vi "Read Device ID Type1.vi"(8 "error in (no error)":errorcluster, 11 "device data model in":refnum<class "Standard Data Model1.lvclass">) -> (0 "error out":errorcluster, 2 "read device ID code":u8(ring)=1 items=["None"=0, "Basic Stream"=1, "Regular Stream"=2, "Extended Stream"=3, "Basic Stream/Individual"=129, "Regular Stream/Individual"=130, "Extended Stream/Individual"=131], 3 "device data model out":refnum<class "Standard Data Model1.lvclass">)   [LabVIEW 2019, in "NI_modbus_upd.lvlib" / "Standard Data Model1.lvclass"]
doc: "Reads the device ID stored in the device data model."
uses:
  Standard Data Model1.lvclass
  Standard Data Model1.lvclass/Standard Data Model1.ctl
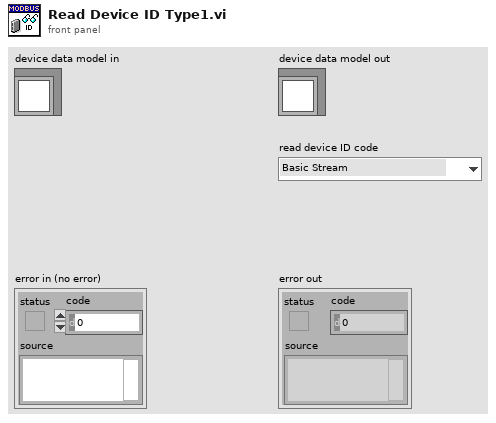
[diagram p1: front panel]
types:
  T1 = typedef "Device ID Type1.ctl" = u8
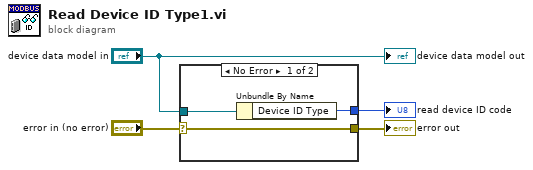
[diagram p0: block diagram]
diagram:
  n1 = case shown="No Error" "error in (no error)" {
    selector: "error in (no error)" -> [w5 w8]
    tunnel: "device data model in" -> [w7 _]
    tunnel: [w6 _] -> w3
    tunnel: [w5 w8] -> w1
    frame No Error {
      n2 = Unbundle By Name(w7) -> ("Device ID Type"=w6:T1)
    }
    frame Error {
    }
  }
  "error out" <- w1
  "read device ID code" <- w3
  "device data model out" <- "device data model in"
